vi "fgt set sensor Regulation Inverted.vi"(8 "error in (no error)":errorcluster, 10 "inverted":bool, 11 "sensorIndex":u32) -> (0 "error out":errorcluster)   [LabVIEW 2016, in "fgt_SDK.lvlib"]
doc: "Specify whether the sensor is inverted in the physical setup, i.e., if an increase in pressure causes the sensor value to decrease and vice-versa."
uses:
  fgt_SDK.lvlib
  dlls/fgt_SDK_32.dll
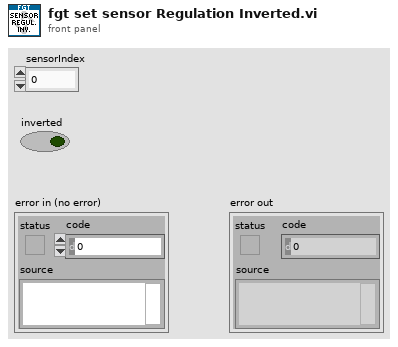
[diagram p1: front panel]
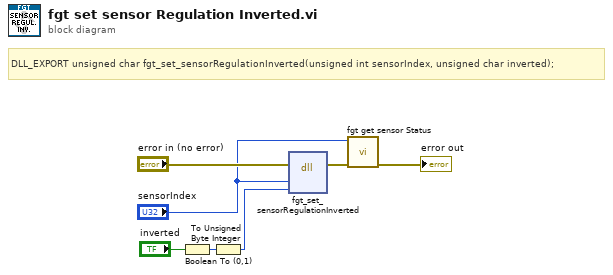
[diagram p0: block diagram]
diagram:
  # "DLL_EXPORT unsigned char fgt_set_sensorRegulationInverted(unsigned int sensorIndex, unsigned char inverted);"
  n1 = Boolean To (0,1)(Boolean="inverted") -> (0, 1=w3:i16)
  n2 = To Unsigned Byte Integer(number=w3) -> (unsigned 8bit integer=w1:u8)
  n3 = dll-call lib="C:/projects/SDK/fgt-SDK-source/bindings/LabVIEW/dlls/fgt_SDK_*.*" fn="fgt_set_sensorRegulationInverted"(error in="error in (no error)", "sensorIndex"="sensorIndex", "inverted"=w1) -> (error out=w6:errorcluster)  [unwired: 5 in, 1 out]
  n4 = call "fgt get sensor Status.vi"("error in (no error)"=w6, "pressureIndex"="sensorIndex") -> ("error out"=→"error out":errorcluster)  [unwired: 9 in]
